vi "CryoTempVoltToKelvin.vi"(10 "CryoTemp calibration":path, 11 "Cryo temp [V]":dbl) -> (0 "Y":dbl[](array[numeric]), 1 "X":dbl[](array[numeric]), 2 "Comment":string, 3 "Cryotemp [K]":dbl)   [LabVIEW 2014]
uses:
  <vilib>/Utility/file.llb/Read From Spreadsheet File (DBL).vi
  <vilib>/Utility/file.llb/Read From Spreadsheet File (string).vi
  <vilib>/gmath/NI_Gmath.lvlib
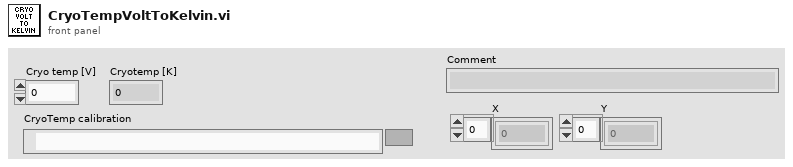
[diagram p1: front panel]
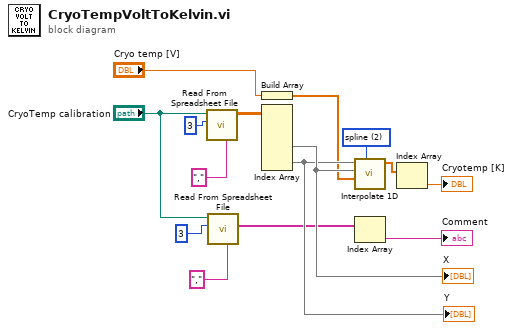
[diagram p0: block diagram]
diagram:
  w14 = 2 items=["nearest", "linear", "spline", "cubic Hermite", "Lagrange"] ("method")
  n1 = call-poly <vilib>:"Read From Spreadsheet File.vi"("delimiter (\\t)"="," ("delimiter (\\t)"), "number of rows (all:-1)"=3, "file path (dialog if empty)"="CryoTemp calibration") -> ("all rows"=w11:dbl[][])  [unwired: 4 in, 4 out]
  n2 = call-poly <vilib>:"Read From Spreadsheet File.vi"("delimiter (\\t)"="," ("delimiter (\\t)"), "number of rows (all:-1)"=3, "file path (dialog if empty)"="CryoTemp calibration") -> ("first row"=w2:string[])  [unwired: 4 in, 4 out]
  n3 = Build Array("Cryo temp [V]") -> (w6:dbl[])
  n4 = Index Array(array=w11) -> (element #2=w13:dbl[], element #3=w12:dbl[])  [unwired: 6 in, 1 out]
  "Y" <- w12
  "X" <- w13
  n5 = call <vilib>:"Interpolate 1D.vi"("method"=w14, "xi"=w6, "X"=w13, "Y"=w12) -> ("yi"=w15:dbl[])  [unwired: 5 in, 2 out]
  n6 = Index Array(array=w2) -> (element=→"Comment":string)  [unwired: 1 in]
  n7 = Index Array(array=w15) -> (element=→"Cryotemp [K]":dbl)  [unwired: 1 in]
